vi "xdata_write.vi"(5 "COM":bool, 7 "VISA name":refnum<visa-resource-name>, 9 "data":u8[](array[numeric]), 10 "wLen":u16, 11 "wAddr":u16) -> (3 "return":i32)   [LabVIEW 2016]
panel:
  in  "vd_cmd_short_header_t":T1
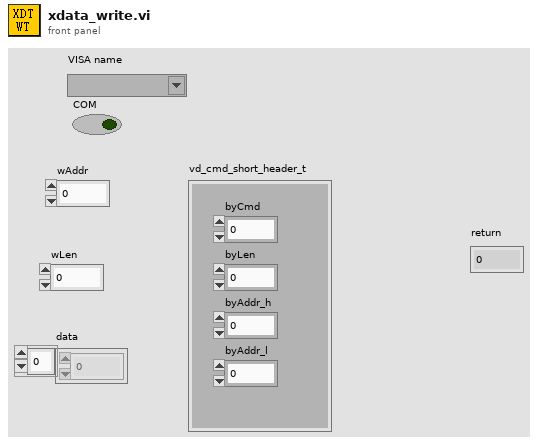
[diagram p1: front panel]
types:
  T1 = cluster{"byCmd":u8, "byLen":u8, "byAddr_h":u8, "byAddr_l":u8}
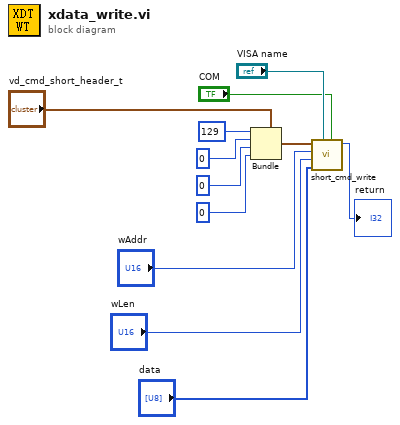
[diagram p0: block diagram]
diagram:
  n1 = Bundle(cluster="vd_cmd_short_header_t", "byCmd"=u8 129, "byLen"=u8 0, "byAddr_h"=u8 0, "byAddr_l"=u8 0) -> (w7:T1)
  n2 = call "short_cmd_write.vi"("COM"="COM", "VISA name"="VISA name", "data"="data", "dwLen"="wLen", "dwAddr"="wAddr", "cmd_short_header_t"=w7) -> ("return"=→"return":i32)  [unwired: 5 in]
